vi "GetReadingRequest.vi"(8 "error in (no error)":errorcluster, 11 "ModuleID":i32) -> (0 "error out":errorcluster)   [LabVIEW 2014, in "SamplerPlugins.lvlib" / "SamplerPluginsBase.lvclass"]
uses:
  SamplerPluginsBase.lvclass
  SamplerModule/Protected/clEventType.ctl
  <vilib>/Utility/error.llb/Error Cluster From Error Code.vi
  <vilib>/ErrorRing/Error Ring.xnode
  SamplerModule/SamplerModule.lvlib
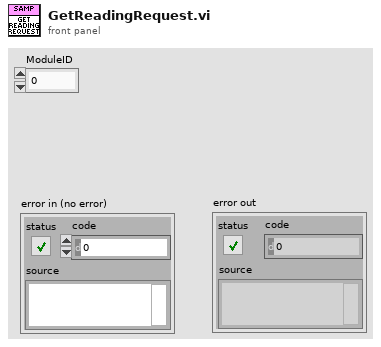
[diagram p1: front panel]
types:
  T1 = typedef "SamplerModule.lvlib/clRequestEvents.ctl" = cluster{"StopRequest":refnum<user-event>, "PathToINI":refnum<user-event>, " LoadPlugin":refnum<user-event>, "ConfigMeasurement":refnum<user-event>, "Read":refnum<user-event>, "GetReading":refnum<user-event>, "InitializeDevice":refnum<user-event>, "ResetRequest":refnum<user-event>, "AbortRequest":refnum<user-event>, "FetchRequest":refnum<user-event>, "InitiateRequest":refnum<user-event>, "ConfigTrigger":refnum<user-event>, "IsOverRange":refnum<user-event>, "ConfigACBandwidth":refnum<user-event>, "ConfigFreqVoltRange":refnum<user-event>, "ConfigMeasCompDest":refnum<user-event>, "FetchMultiPoint":refnum<user-event>, "ReadMultiPoint":refnum<user-event>, "ConfigMultiPoint":refnum<user-event>, "GetMultiPointReading":refnum<user-event>, "InitiateMultiPoint":refnum<user-event>}
  T2 = typedef "SamplerModule.lvlib/clEventType.ctl" = cluster{"ModuleID":i32, "Data":variant}
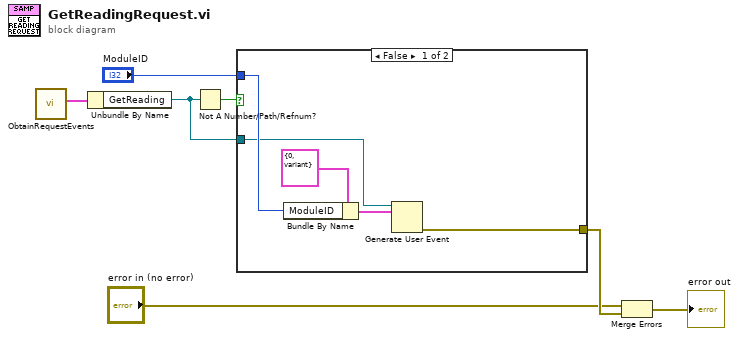
[diagram p0: block diagram]
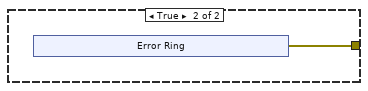
[diagram p2: hidden frame]
diagram:
  n1 = call "ObtainRequestEvents.vi"() -> ("SamplerRequests"=w7:T1)  [unwired: 10 in, 1 out]
  n2 = Unbundle By Name(w7) -> ("GetReading"=w5:refnum<user-event>)
  n3 = Not A Number/Path/Refnum?(number/path/refnum=w5) -> (NaN/Path/Refnum?=w6:bool)
  n4 = case shown="False" w6 {
    tunnel: w5 -> [w9 _]
    tunnel: "ModuleID" -> [w11 _]
    tunnel: [w8 w13] -> w2
    frame False {
      n5 = Bundle By Name(cluster=T2 {"ModuleID"=0, "Data"=variant} ("clEventType"), "ModuleID"=w11) -> (w10:T2)
      n6 = Generate User Event(user event=w9, event data cluster=w10) -> (error out=w8:errorcluster)  [unwired: 2 in, 1 out]
    }
    frame True {
      n7 = xnode "Error Ring"() -> ("error out"=w13:errorcluster)
    }
  }
  n8 = Merge Errors("error in (no error)", w2) -> (→"error out":errorcluster)
